vi "Example Read Write String Data.vi"() -> ()   [LabVIEW 2019, in "D2XX-lv.lvlib"]
uses:
  D2XX-lv.lvlib
  D2XX_Functions_7.0/FT_Open_Device_By_Serial_Number.vi
  private/FT_Status to Error.vi
  private/Read Data (String).vi
  private/Write Data (String).vi
  private/Open Device (Serial Number).vi
panel:
  out "Read Buffer":string
  in  "Write Buffer":string
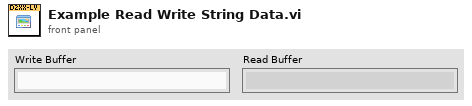
[diagram p1: front panel]
types:
  T1 = cluster{"Word Length":u8, "Stop Bits":u8, "Parity":u8}
  T2 = typedef "D2XX-lv.lvlib/Device Info.ctl" = cluster{"Serial Number":string, "COM port":string, "Description":string}
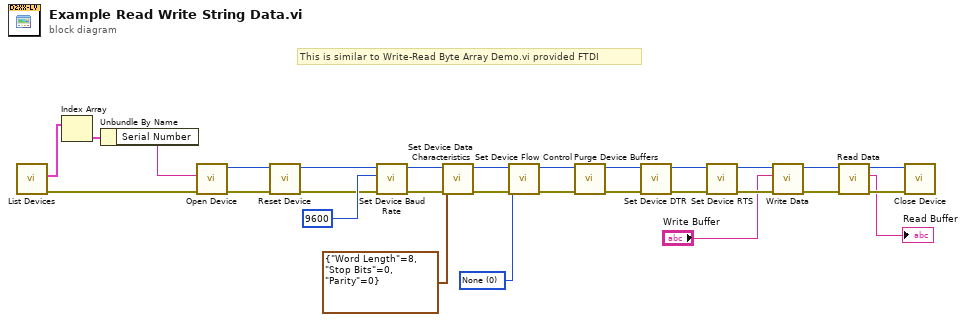
[diagram p0: block diagram]
diagram:
  w11 = u16 0 items=["None"=0, "RTS-CTS"=256, "DTR-DSR"=512, "XOn-XOff"=1024] ("Flow Control")
  # "This is similar to Write-Read Byte Array Demo.vi provided FTDI"
  n1 = call "List Devices.vi"() -> ("error out"=w7:errorcluster, "Devices"=w8:T2[])  [unwired: 10 in]
  n2 = Index Array(array=w8) -> (element=w6:T2)  [unwired: 1 in]
  n3 = Unbundle By Name(w6) -> ("Serial Number"=w5:string)
  n4 = call-poly "Open Device.vi"("error in (no error)"=w7, "Device Serial Number"=w5) -> ("error out"=w4:errorcluster, "Handle"=w3:u32)  [unwired: 8 in]
  n5 = call "Reset Device.vi"("error in (no error)"=w4, "Handle"=w3) -> ("error out"=w1:errorcluster, "Handle out"=w2:u32)  [unwired: 8 in]
  n6 = call "Set Device Baud Rate.vi"("error in (no error)"=w1, "Baud Rate"=u32 9600, "Handle"=w2) -> ("error out"=w28:errorcluster, "Handle out"=w29:u32)  [unwired: 7 in]
  n7 = call "Set Device Data Characteristics.vi"("error in (no error)"=w28, "Data Characteristics"=T1 {"Word Length"=8, "Stop Bits"=0, "Parity"=0}, "Handle"=w29) -> ("error out"=w26:errorcluster, "Handle out"=w27:u32)  [unwired: 7 in]
  n8 = call "Set Device Flow Control.vi"("error in (no error)"=w26, "Flow Control"=w11, "Handle"=w27) -> ("error out"=w24:errorcluster, "Handle out"=w25:u32)  [unwired: 7 in]
  n9 = call "Purge Device Buffers.vi"("error in (no error)"=w24, "Handle"=w25) -> ("error out"=w22:errorcluster, "Handle out"=w23:u32)  [unwired: 8 in]
  n10 = call "Set Device DTR.vi"("error in (no error)"=w22, "Handle"=w23) -> ("error out"=w20:errorcluster, "Handle out"=w21:u32)  [unwired: 8 in]
  n11 = call "Set Device RTS.vi"("error in (no error)"=w20, "Handle"=w21) -> ("error out"=w18:errorcluster, "Handle out"=w19:u32)  [unwired: 8 in]
  n12 = call-poly "Write Data.vi"("error in (no error)"=w18, "Write Buffer"="Write Buffer", "Handle"=w19) -> ("error out"=w16:errorcluster, "Handle out"=w17:u32)  [unwired: 6 in, 1 out]
  n13 = call-poly "Read Data.vi"("error in (no error)"=w16, "Handle"=w17) -> ("error out"=w14:errorcluster, "Read Buffer"=→"Read Buffer":string, "Handle out"=w15:u32)  [unwired: 6 in, 1 out]
  n14 = call "Close Device.vi"("error in (no error)"=w14, "Handle"=w15) -> ()  [unwired: 9 in, 1 out]
